vi "Extrae_ScanTemp.vi"(10 "T string":string="Scan Temp from 20K to 100K at 0.1K/min, in 6 steps, Uniform, Vuelta") -> (1 "Array T":string[](array[string]))   [LabVIEW 2017]
panel:
  out "Vuelta":bool
  # "Set Temperatura 4.2K at 20K/min, FastSettle"
  # "Scan Temp from 20K to 200K at 0.1K/min, in 50 steps, Uniform, Vuelta"
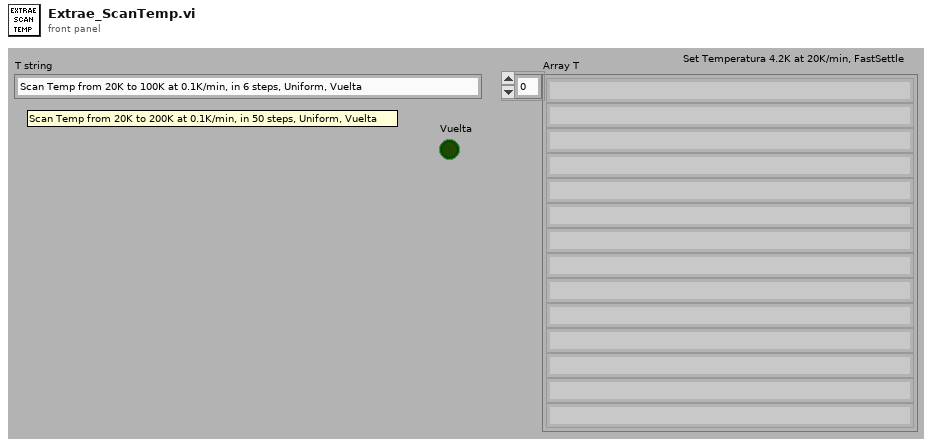
[diagram p1: front panel]
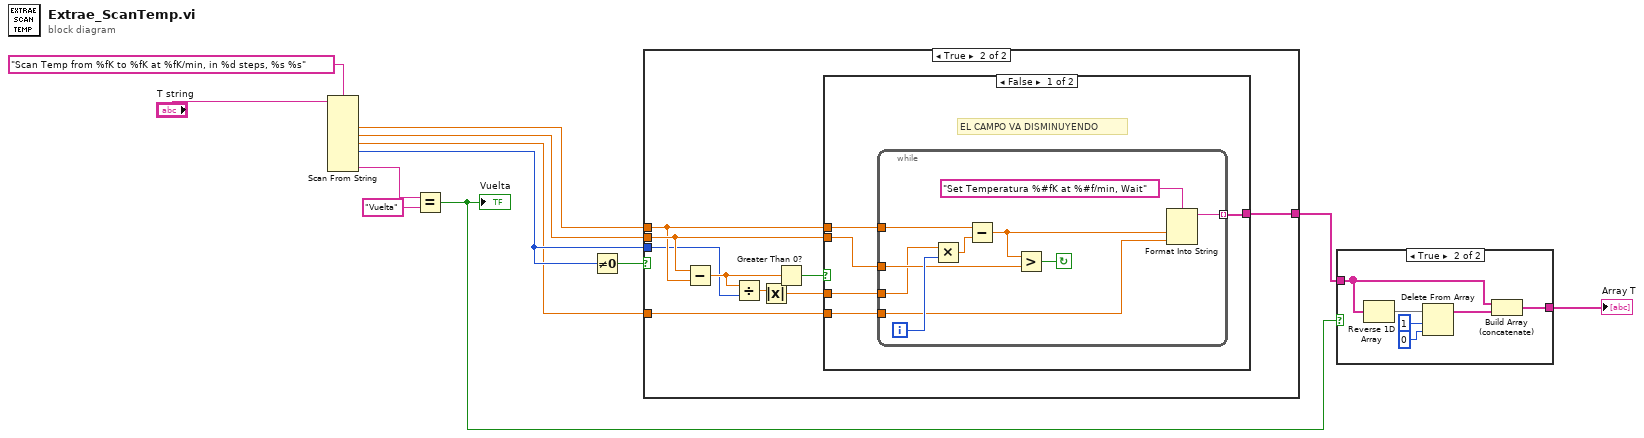
[diagram p0: block diagram]
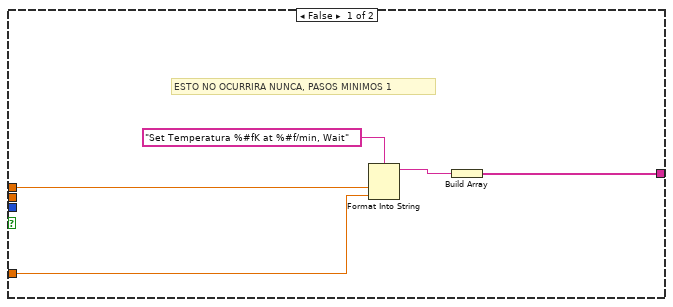
[diagram p3: hidden frame]
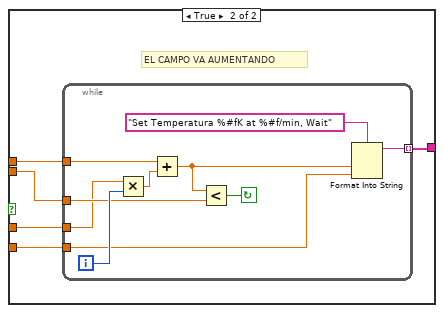
[diagram p4: hidden frame]
diagram:
  n1 = Scan From String(format string="Scan Temp from %fK to %fK at %fK/min, in %d steps, %s %s", input string="T string") -> (output 1=w9:dbl, output 2=w8:dbl, output 3=w6:dbl, output 4=w7:i32, output 6=w1:string)  [unwired: 9 in, 3 out]
  n2 = Equal?(x=w1, y="Vuelta") -> (x = y?=w3:bool)
  "Vuelta" <- w3
  n3 = Not Equal To 0?(x=w7) -> (x != 0?=w10:bool)
  n4 = case shown="True" w10 {
    tunnel: w8 -> [_ w25]
    tunnel: w9 -> [w16 w24]
    tunnel: w7 -> [_ w20]
    tunnel: w6 -> [w15 w23]
    tunnel: [w13 w22] -> w2
    frame False {
      # "ESTO NO OCURRIRA NUNCA, PASOS MINIMOS 1"
      n5 = Format Into String(format string="Set Temperatura %#fK at %#f/min, Wait", w16, w15) -> (resulting string=w14:string)  [unwired: 2 in, 1 out]
      n6 = Build Array(w14) -> (w13:string[])
    }
    frame True {
      n7 = Subtract(x=w25, y=w24) -> (x-y=w21:dbl)
      n8 = Divide(x=w21, y=w20) -> (x/y=w19:dbl)
      n9 = Absolute Value(x=w19) -> (abs(x)=w18:dbl)
      n10 = Greater Than 0?(x=w21) -> (x > 0?=w26:bool)
      n11 = case shown="False" w26 {
        tunnel: [w28 w43] -> w22
        tunnel: w25 -> [w31 w46]
        tunnel: w24 -> [w30 w45]
        tunnel: w23 -> [w29 w44]
        tunnel: w18 -> [w27 w42]
        frame False {
          # "EL CAMPO VA DISMINUYENDO"
          n12 = while {
            tunnel: w30 -> [w39]
            tunnel: w31 -> [w38]
            tunnel: w29 -> [w35]
            tunnel: [w33] -> w28 mode=indexing
            tunnel: w27 -> [w32]
            i -> [w41]
            stop <- w37 continue-if-true
            n13 = Multiply(x=w32, y=w41) -> (x*y=w40:dbl)
            n14 = Subtract(x=w39, y=w40) -> (x-y=w36:dbl)
            n15 = Greater?(x=w36, y=w38) -> (0:w37:bool)
            n16 = Format Into String(format string="Set Temperatura %#fK at %#f/min, Wait", w36, w35) -> (resulting string=w33:string)  [unwired: 2 in, 1 out]
          }
        }
        frame True {
          # "EL CAMPO VA AUMENTANDO"
          n17 = while {
            tunnel: w45 -> [w54]
            tunnel: w46 -> [w53]
            tunnel: w44 -> [w50]
            tunnel: [w48] -> w43 mode=indexing
            tunnel: w42 -> [w47]
            i -> [w56]
            stop <- w52 continue-if-true
            n18 = Multiply(x=w47, y=w56) -> (x*y=w55:dbl)
            n19 = Add(x=w54, y=w55) -> (x+y=w51:dbl)
            n20 = Less?(x=w51, y=w53) -> (x < y?=w52:bool)
            n21 = Format Into String(format string="Set Temperatura %#fK at %#f/min, Wait", w51, w50) -> (resulting string=w48:string)  [unwired: 2 in, 1 out]
          }
        }
      }
    }
  }
  n22 = case shown="True" w3 {
    tunnel: w2 -> [w57 w58]
    tunnel: [w57 w59] -> w4
    frame False {
    }
    frame True {
      n23 = Reverse 1D Array(array=w58) -> (reversed array=w62:string[])
      n24 = Delete From Array(array=w62, length=1, index=0) -> (array with subset deleted=w60:string[])  [unwired: 1 out]
      n25 = Build Array (concatenate)(w58, w60) -> (w59:string[])
    }
  }
  "Array T" <- w4
